vi "lab6_task3.vi"() -> ()   [LabVIEW 2021]
uses:
  <vilib>/Analysis/1siggen.llb/Ramp Pattern by Samples.vi
  <vilib>/Analysis/NI_AALBase.lvlib
panel:
  out "XY Graph":cluster{"X":dbl, "Y":dbl}[](graph)
  in  "stop":bool
  out "Voltage Output":dbl
  in  "start":dbl format="%0.2f"
  in  "end":dbl=1.0 format="%0.2f"
  out "# Sample":i32
  in  "samples":i32=128
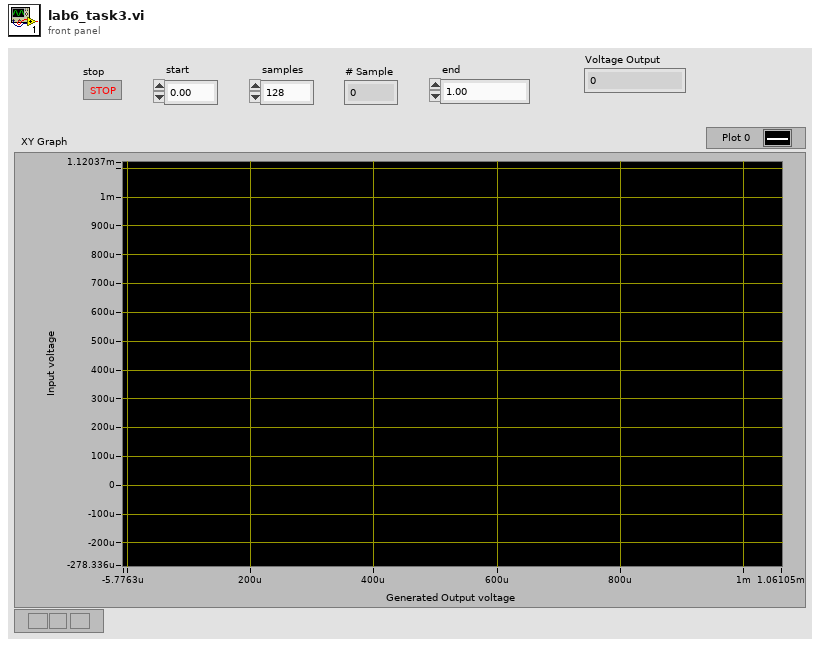
[diagram p1: front panel]
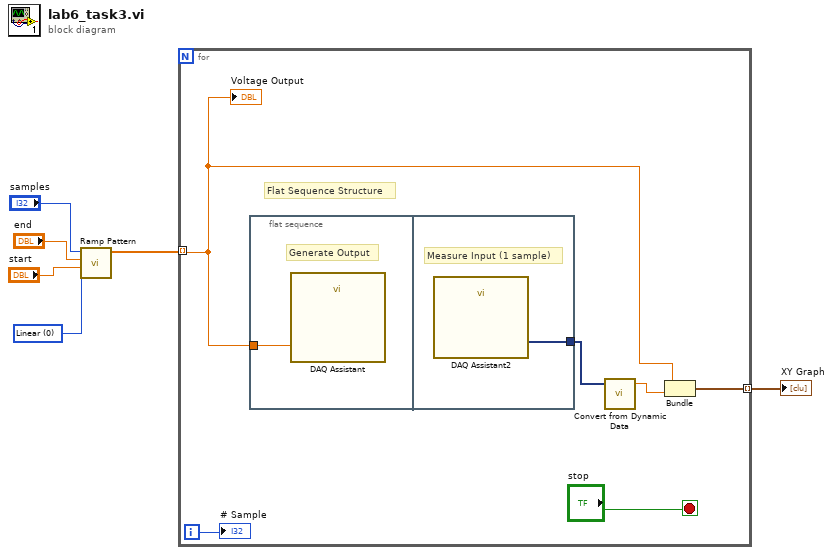
[diagram p0: block diagram]
diagram:
  w3 = u16 0 items=["Linear", "Logarithmic"] ("type")
  n1 = call-poly <vilib>:"Ramp Pattern.vi"("type"=w3, "start"="start", "end"="end", "samples"="samples") -> ("Ramp Pattern"=w2:dbl[])  [unwired: 6 in, 1 out]
  n2 = for {
    tunnel: w2 -> [w9] mode=indexing
    tunnel: [w7] -> w1 mode=indexing
    i -> [w12]
    stop <- "stop" stop-if-true
    # "Flat Sequence Structure"
    n3 = flat-sequence {
      tunnel: w9 -> [w13]
      tunnel: [w14] -> w11
      frame #0 {
        # "Generate Output"
        n4 = call "DAQ Assistant"("data"=w13) -> ()  [unwired: 17 in, 2 out]
      }
      frame #1 {
        # "Measure Input (1 sample)"
        n5 = call "DAQ Assistant2"() -> ("data"=w14:dynamicdata)  [unwired: 17 in, 2 out]
      }
    }
    n6 = call "Convert from Dynamic Data"("Dynamic Data Type"=w11) -> ("Scalar"=w10:dbl)  [unwired: 3 in]
    n7 = Bundle(w9, "Scalar"=w10) -> (w7:cluster{dbl, "Scalar":dbl})  [unwired: 1 in]
    "# Sample" <- w12
    "Voltage Output" <- w9
  }
  "XY Graph" <- w1
